vi "digidatadaq.vi"() -> ()   [LabVIEW 2018]
panel:
  in  "rate":dbl=1000.0
  in  "data":digitalwaveform[](array[waveform])
  in  "stop (F)":bool
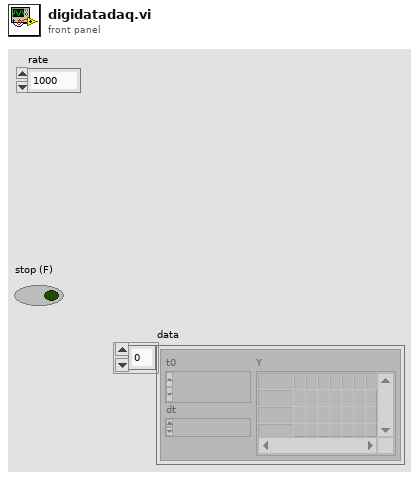
[diagram p1: front panel]
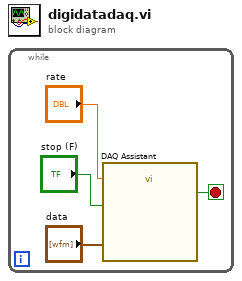
[diagram p0: block diagram]
diagram:
  n1 = while {
    stop <- w4 stop-if-true
    n2 = call "DAQ Assistant"("data"="data", "rate"="rate", "stop (F)"="stop (F)") -> ("stopped"=w4:bool)  [unwired: 14 in, 2 out]
  }
